vi "DB - Replace DB.Schema.Table.vi"(4 "DB.Schema.Table 4":T1, 6 "DB.Schema.Table 3":T1, 7 "DB.Schema.Table 5":T1, 8 "error in (no error)":errorcluster, 9 "DB.Schema.Table 2":T1, 10 "DB.Schema.Table":T1, 11 "string in":string) -> (0 "error out":errorcluster, 3 "string out":string)   [LabVIEW 2020]
uses:
  Control/DB - DB.Schema.Table.ctl
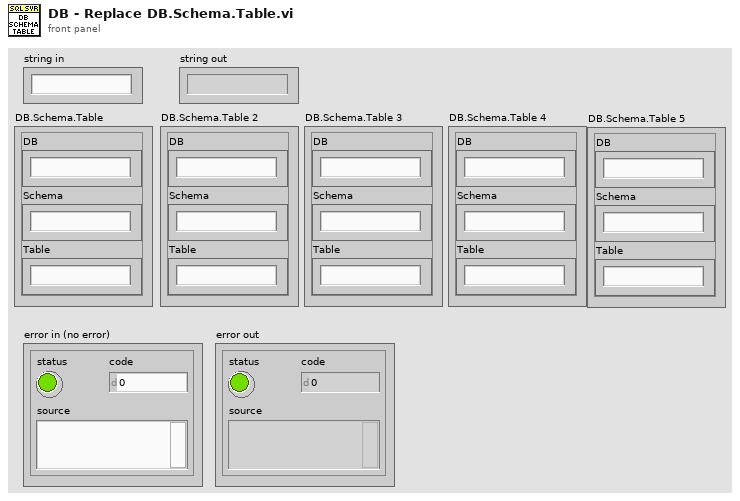
[diagram p1: front panel]
types:
  T1 = typedef "DB - DB.Schema.Table.ctl" = cluster{"DB":string, "Schema":string, "Table":string}
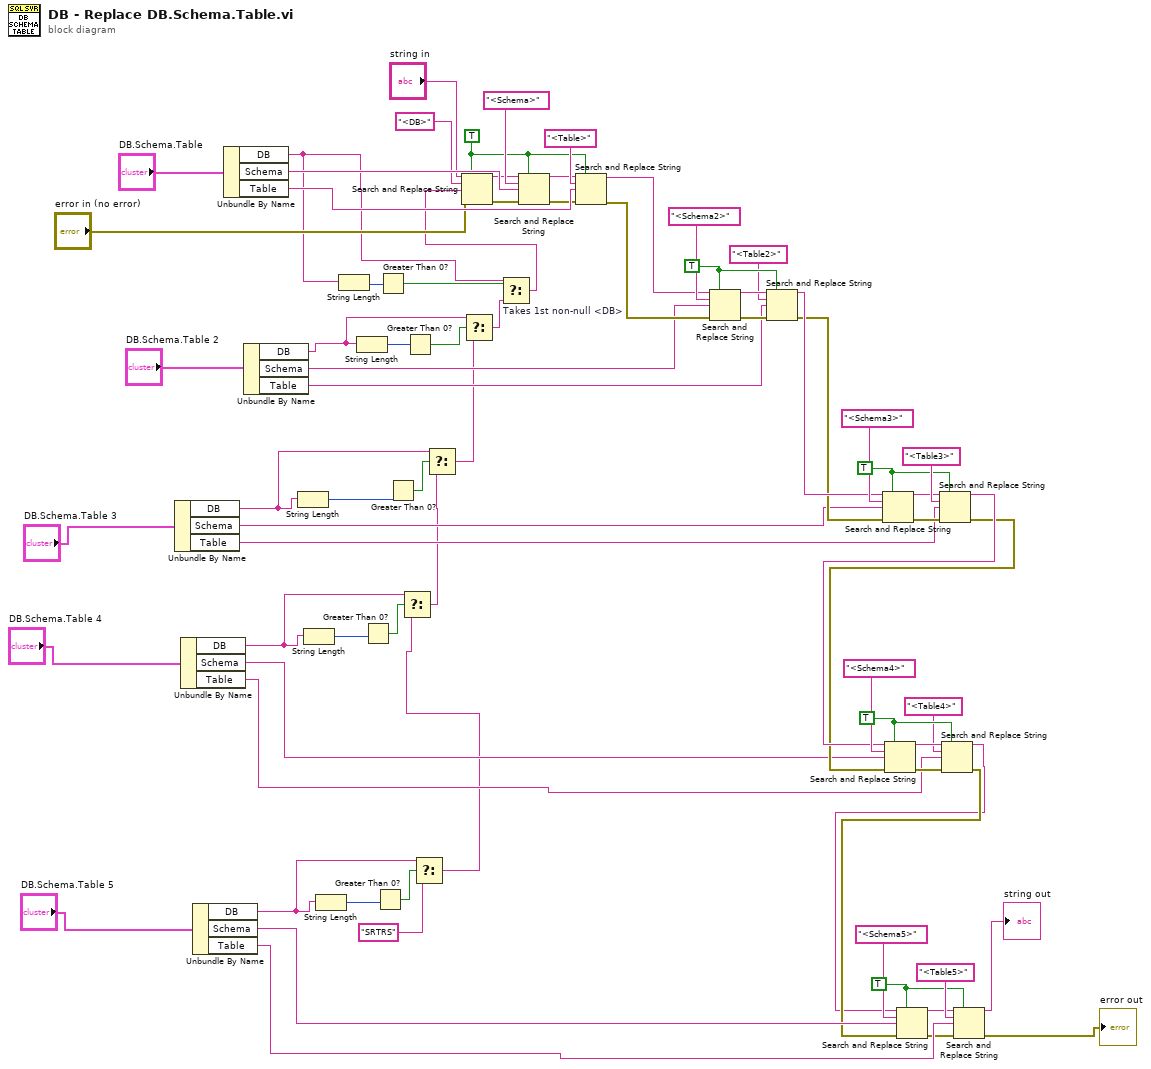
[diagram p0: block diagram]
diagram:
  w11 = TRUE ("replace all? (F)")
  w27 = TRUE ("replace all? (F)")
  w49 = TRUE ("replace all? (F)")
  w63 = TRUE ("replace all? (F)")
  w64 = TRUE ("replace all? (F)")
  n1 = Unbundle By Name("DB.Schema.Table 3") -> ("DB"=w34:string, "Schema"=w46:string, "Table"=w44:string)
  n2 = Unbundle By Name("DB.Schema.Table 4") -> ("DB"=w31:string, "Schema"=w20:string, "Table"=w19:string)
  n3 = Unbundle By Name("DB.Schema.Table 5") -> ("DB"=w7:string, "Schema"=w16:string, "Table"=w17:string)
  n4 = Unbundle By Name("DB.Schema.Table") -> ("DB"=w41:string, "Schema"=w75:string, "Table"=w76:string)
  n5 = Unbundle By Name("DB.Schema.Table 2") -> ("DB"=w37:string, "Schema"=w55:string, "Table"=w54:string)
  n6 = String Length(string=w34) -> (length=w38:i32)
  n7 = String Length(string=w31) -> (length=w29:i32)
  n8 = String Length(string=w7) -> (length=w9:i32)
  n9 = String Length(string=w41) -> (length=w43:i32)
  n10 = String Length(string=w37) -> (length=w40:i32)
  n11 = Greater Than 0?(x=w29) -> (x > 0?=w30:bool)
  n12 = Greater Than 0?(x=w9) -> (x > 0?=w8:bool)
  n13 = Greater Than 0?(x=w43) -> (x > 0?=w42:bool)
  n14 = Greater Than 0?(x=w38) -> (x > 0?=w35:bool)
  n15 = Greater Than 0?(x=w40) -> (x > 0?=w39:bool)
  n16 = Select(t=w7, s=w8, f="SRTRS") -> (s? t:f=w1:string)
  n17 = Select(t=w31, s=w30, f=w1) -> (s? t:f=w18:string)
  n18 = Select(t=w34, s=w35, f=w18) -> (s? t:f=w33:string)
  n19 = Select(t=w37, s=w39, f=w33) -> (s? t:f=w36:string)
  n20 = Select "Takes 1st non-null <DB>"(t=w41, s=w42, f=w36) -> (s? t:f=w32:string)
  n21 = Search and Replace String(replace all?=w64, input string="string in", search string="<DB>", replace string=w32, error in="error in (no error)") -> (result string=w71:string, error out=w67:errorcluster)  [unwired: 3 in, 2 out]
  n22 = Search and Replace String(replace all?=w64, input string=w71, search string="<Schema>", replace string=w75, error in=w67) -> (result string=w72:string, error out=w66:errorcluster)  [unwired: 3 in, 2 out]
  n23 = Search and Replace String(replace all?=w64, input string=w72, search string="<Table>", replace string=w76, error in=w66) -> (result string=w57:string, error out=w58:errorcluster)  [unwired: 3 in, 2 out]
  n24 = Search and Replace String(replace all?=w63, input string=w57, search string="<Schema2>", replace string=w55, error in=w58) -> (result string=w61:string, error out=w62:errorcluster)  [unwired: 3 in, 2 out]
  n25 = Search and Replace String(replace all?=w63, input string=w61, search string="<Table2>", replace string=w54, error in=w62) -> (result string=w48:string, error out=w47:errorcluster)  [unwired: 3 in, 2 out]
  n26 = Search and Replace String(replace all?=w49, input string=w48, search string="<Schema3>", replace string=w46, error in=w47) -> (result string=w51:string, error out=w50:errorcluster)  [unwired: 3 in, 2 out]
  n27 = Search and Replace String(replace all?=w49, input string=w51, search string="<Table3>", replace string=w44, error in=w50) -> (result string=w22:string, error out=w21:errorcluster)  [unwired: 3 in, 2 out]
  n28 = Search and Replace String(replace all?=w27, input string=w22, search string="<Schema4>", replace string=w20, error in=w21) -> (result string=w25:string, error out=w26:errorcluster)  [unwired: 3 in, 2 out]
  n29 = Search and Replace String(replace all?=w27, input string=w25, search string="<Table4>", replace string=w19, error in=w26) -> (result string=w3:string, error out=w4:errorcluster)  [unwired: 3 in, 2 out]
  n30 = Search and Replace String(replace all?=w11, input string=w3, search string="<Schema5>", replace string=w16, error in=w4) -> (result string=w13:string, error out=w12:errorcluster)  [unwired: 3 in, 2 out]
  n31 = Search and Replace String(replace all?=w11, input string=w13, search string="<Table5>", replace string=w17, error in=w12) -> (result string=→"string out":string, error out=→"error out":errorcluster)  [unwired: 3 in, 2 out]
